vi "Add Waveform to Chart.vi"(8 "error in (no error)":errorcluster, 10 "Waveform In":waveform(dbl), 11 "Chart Actor in":refnum<class "Chart Actor.lvclass">) -> (0 "error out":errorcluster, 3 "Chart Actor out":refnum<class "Chart Actor.lvclass">)   [LabVIEW 2021, in "Chart Actor.lvlib" / "Chart Actor.lvclass"]
uses:
  Chart Actor.lvclass
  Chart Actor.lvclass/Chart Actor.ctl
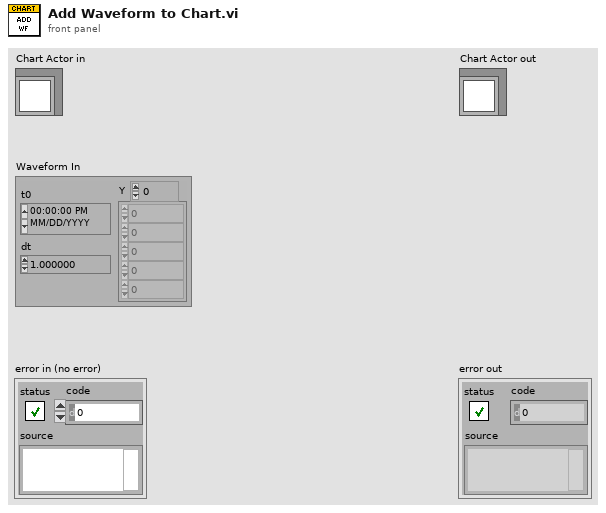
[diagram p1: front panel]
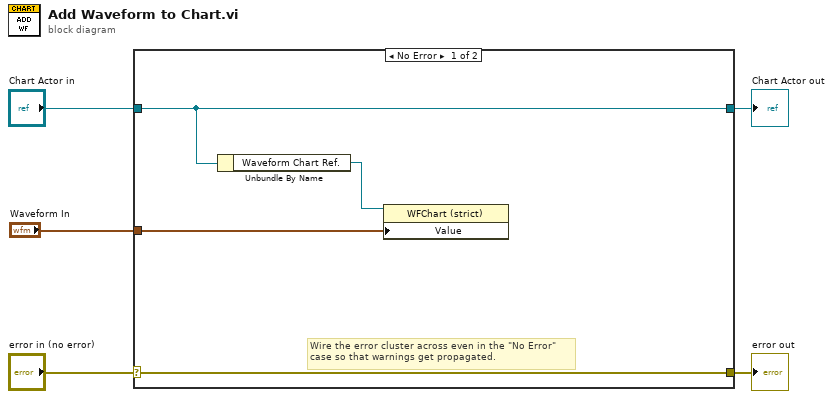
[diagram p0: block diagram]
diagram:
  n1 = case shown="No Error" "error in (no error)" {
    selector: "error in (no error)" -> [w9 w11]
    tunnel: [w9 w11] -> w4
    tunnel: [w8 w10] -> w2
    tunnel: "Chart Actor in" -> [w8 w10]
    tunnel: "Waveform In" -> [w6 _]
    frame No Error {
      # "Wire the error cluster across even in the \"No Error\"\ncase so that warnings get propagated."
      n2 = Unbundle By Name(w8) -> ("Waveform Chart Ref."=w7:refnum<vi>)
      n3 = property class="WFChart (strict)"(reference=w7, "Value"=w6) -> ()  [unwired: 1 in, 2 out]
    }
    frame Error {
    }
  }
  "error out" <- w4
  "Chart Actor out" <- w2
